vi "decrementMonth.vi"(8 "error in (no error)":errorcluster, 11 "MonthDisplay in":refnum<class "DateUserInterface.lvclass">) -> (0 "error out":errorcluster, 3 "MonthDisplay out":refnum<class "DateUserInterface.lvclass">)   [LabVIEW 2018, in "DateUserInterface.lvclass"]
uses:
  DateUserInterface.lvclass
  DateUserInterface.lvclass/DateUserInterface.ctl
  month.ctl
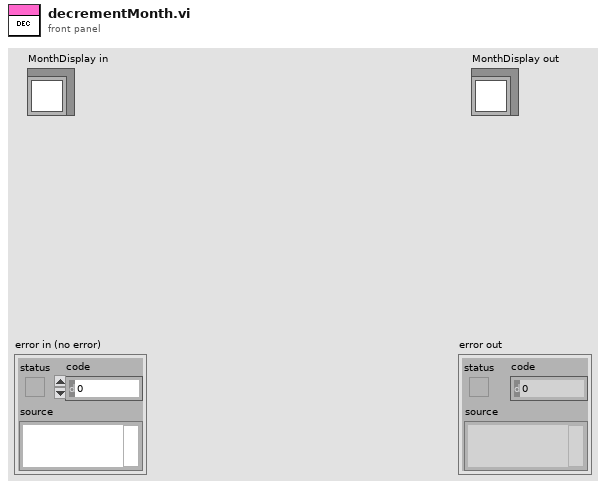
[diagram p1: front panel]
types:
  T1 = typedef "DateUserInterface.lvclass/month.ctl" = enum16{"January", "February", "March", "April", "May", "June", "July", "August", "September", "October", "November", "December"}
  T2 = typedef "MonthDisplay.lvclass/month.ctl" = enum16{"January", "February", "March", "April", "May", "June", "July", "August", "September", "October", "November", "December"}
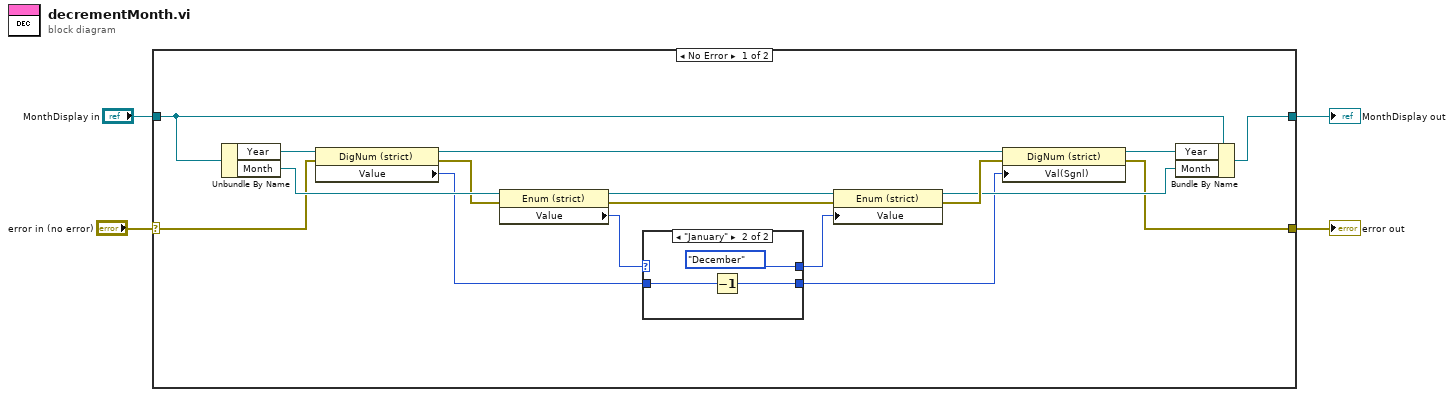
[diagram p0: block diagram]
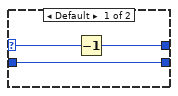
[diagram p2: hidden frame]
diagram:
  n1 = case shown="No Error" "error in (no error)" {
    selector: "error in (no error)" -> [w17 w29]
    tunnel: [w9 w29] -> w1
    tunnel: "MonthDisplay in" -> [w21 w28]
    tunnel: [w20 w28] -> w2
    frame No Error {
      n2 = Unbundle By Name(w21) -> ("Year"=w19:refnum<vi>, "Month"=w18:refnum<vi>)
      n3 = property class="DigNum (strict)"(reference=w19, error in=w17) -> (reference out=w14:refnum<vi>, error out=w16:errorcluster, "Value"=w7:i32)
      n4 = property class="Enum (strict)"(reference=w18, error in=w16) -> (reference out=w12:refnum<vi>, error out=w13:errorcluster, "Value"=w8:T2)
      n5 = case shown="\"January\"" w8 {
        selector: w8 -> [w24 _]
        tunnel: [w22 w27] -> w6
        tunnel: [w23 month."December" ("Month")] -> w5
        tunnel: w7 -> [w22 w26]
        frame Default {
          n6 = Decrement(x=w24) -> (x-1=w23:T2)
        }
        frame "January" {
          n7 = Decrement(x=w26) -> (x-1=w27:i32)
        }
      }
      n8 = property class="Enum (strict)"(reference=w12, error in=w13, "Value"=w5) -> (reference out=w10:refnum<vi>, error out=w11:errorcluster)
      n9 = property class="DigNum (strict)"(reference=w14, error in=w11, "Val(Sgnl)"=w6) -> (reference out=w15:refnum<vi>, error out=w9:errorcluster)
      n10 = Bundle By Name(cluster=w21, "Year"=w15, "Month"=w10) -> (w20:refnum<class "DateUserInterface.lvclass">)
    }
    frame Error {
    }
  }
  "error out" <- w1
  "MonthDisplay out" <- w2
